vi "MCL Monitor Z.vi"(10 "handle":i32, 11 "position":dbl) -> (3 "function return":dbl)   [LabVIEW 2017, in "Madlib.lvlib"]
doc: "MADLIB_API double MCL_MonitorZ(double position, int handle);"
uses:
  Madlib.lvlib
  Madlib.dll
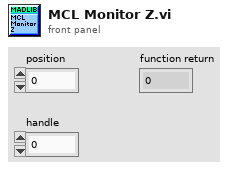
[diagram p1: front panel]
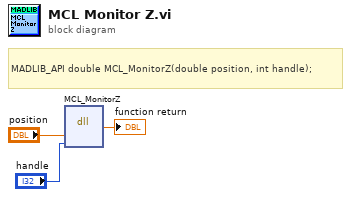
[diagram p0: block diagram]
diagram:
  # "MADLIB_API\tdouble\tMCL_MonitorZ(double position, int handle);"
  n1 = dll-call lib="C:/Users/francesco/dev/pump-probe/Piezo/lvlib/Madlib.*" fn="MCL_MonitorZ"("position"="position", "handle"="handle") -> (→"function return":dbl)  [unwired: 5 in, 2 out]
